vi "Kernel.vi"(0 "reference in":refnum<class "G#Object.lvclass">, 1 "object name":string, 2 "option 1":bool, 3 "option 2":bool, 4 "depth":i32, 5 "error in (no error)":errorcluster, 6 "state":T2, 7 "option 3":bool, 8 "attributes in":variant[](array[variant]), 10 "class attributes in":variant[](array[variant])) -> (11 "class attributes out":variant[](array[variant]), 12 "class hierarchy":T1[](array[typedef]), 13 "attributes out":variant[](array[variant]), 14 "reference out":refnum<class "G#Object.lvclass">, 15 "attribute refs":u32[](array[numeric]), 16 "static attribute ref":u32, 17 "output 1":bool, 18 "output 2":bool, 19 "error out":errorcluster)   [LabVIEW 2017, in "G#Object.lvclass"]
doc: "This is the G#object kernel that is responsible for creating and deleting object."
uses:
  G#Object.lvclass
  utils/G#Object_State.ctl
  utils/G#Object_ClassHierarchy.ctl
  G#Object.lvclass/G#Object.ctl
  utils/G#Object_ObjectInfoType.ctl
  utils/G#Object_CreateMethod.ctl
  utils/G#Object_EventType.ctl
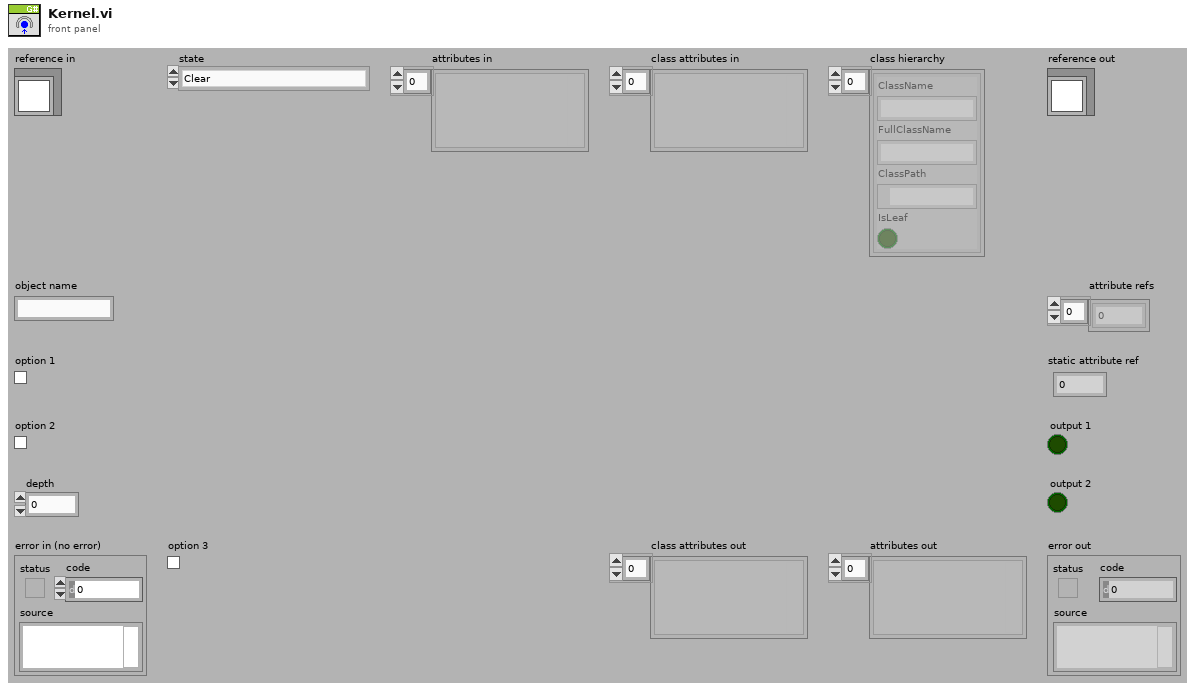
[diagram p1: front panel]
types:
  T1 = typedef "G#Object.lvclass/G#Object_ClassHierarchy.ctl" = cluster{"ClassName":string, "FullClassName":string, "ClassPath":path, "IsLeaf":bool}
  T2 = typedef "G#Object.lvclass/G#Object_State.ctl" = enum16{"Clear", "Create", "Delete", "Get class attributes", "Class hierarchy", "Get attribute value", "Set attribute value"}
  T3 = typedef "G#Object.lvclass/G#Object_ObjectInfoType.ctl" = cluster{"ObjectName":string, "ObjectID":u32, "Users":i32, "Counter":bool, "AttributeRefs":u32[], "FullClassName":string, "ClassName":string, "CreateMethod":T4, "GenericDestructorExists":bool, "Owner":string}
  T4 = typedef "G#Object.lvclass/G#Object_CreateMethod.ctl" = enum16{"Create", "Create or look up existing", "Look up existing"}
  T5 = typedef "G#Object.lvclass/G#Object_EventType.ctl" = enum16{"Created new", "Looked up existing", "Deleted", "Forced delete", "Not deleted", "Garbage collected", "Cleared", "User", "Error", "External create object", "External create class attributes", "Created class attributes", "Run constructor", "Run constructor done", "Run open method", "Run open method done"}
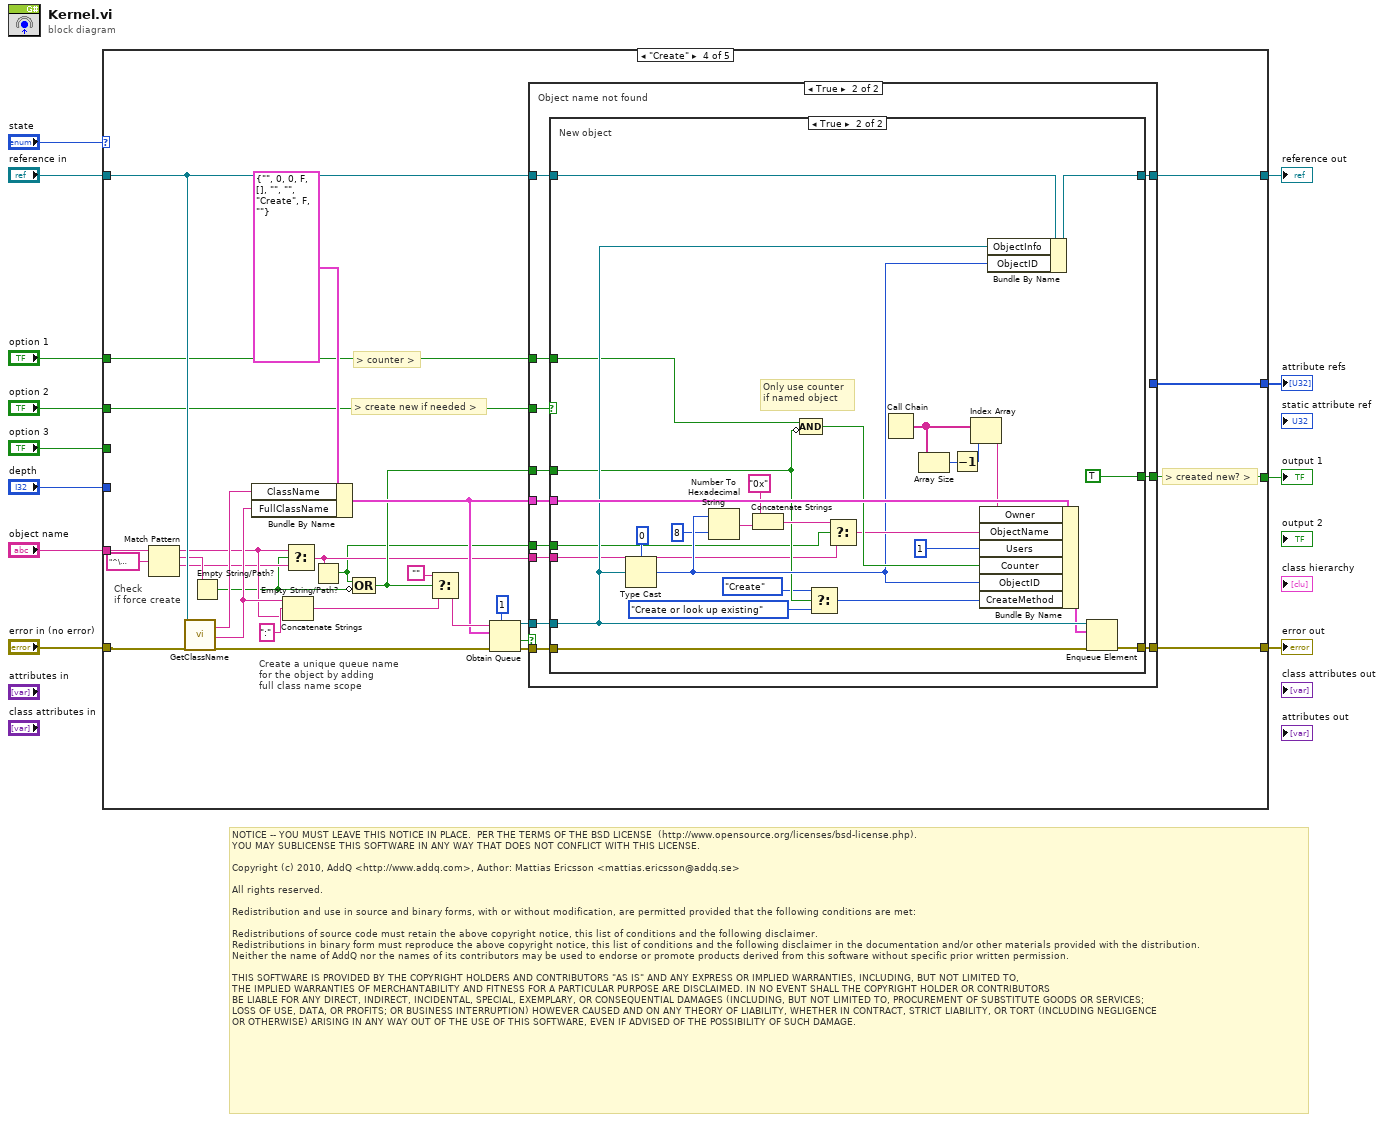
[diagram p0: block diagram]
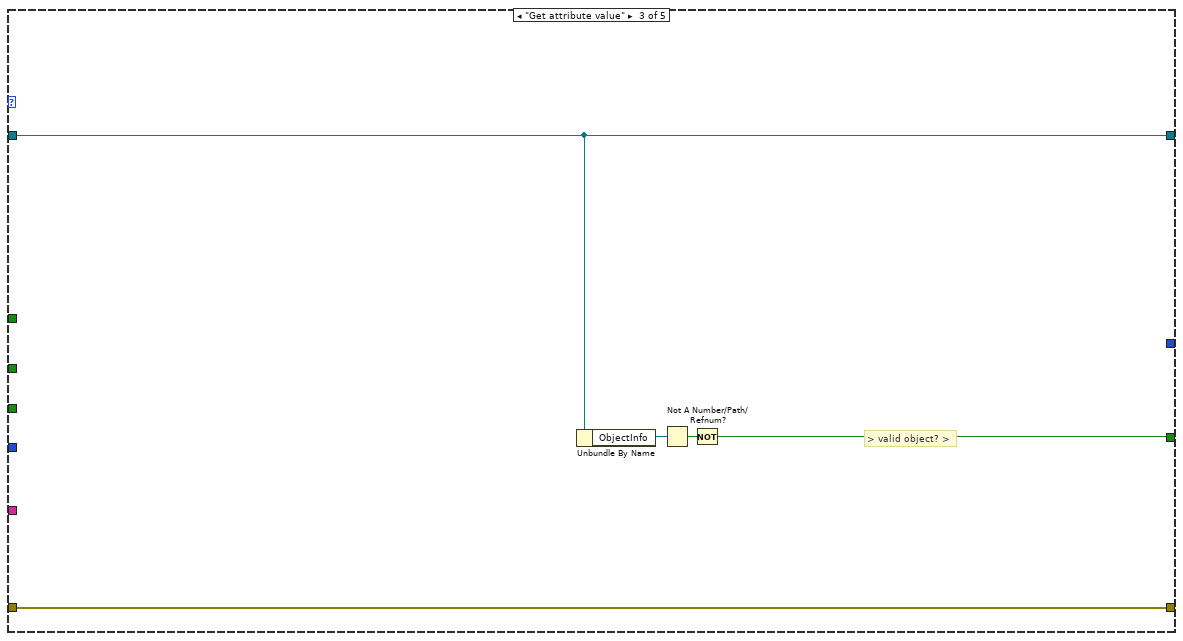
[diagram p4: hidden frame]
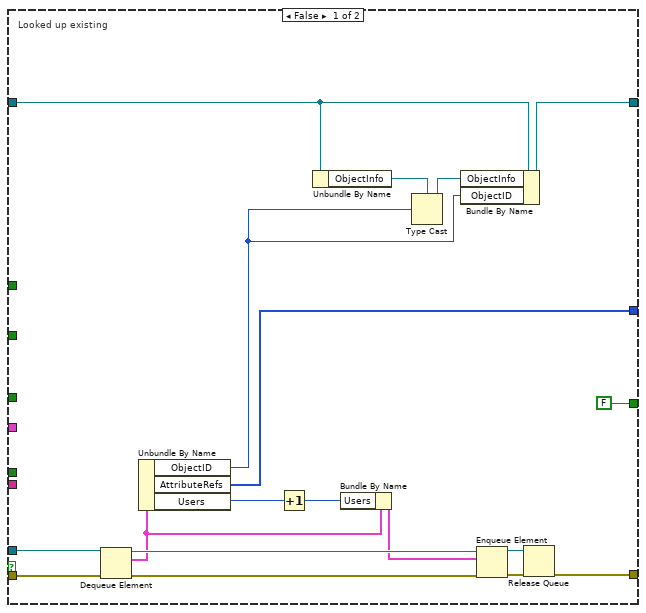
[diagram p5: hidden frame]
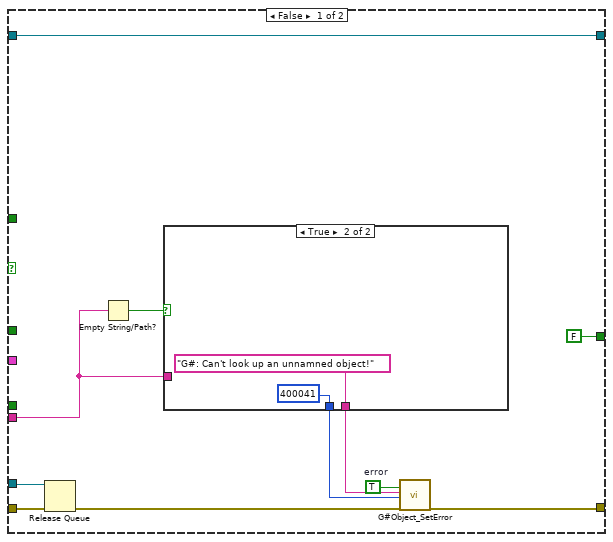
[diagram p6: hidden frame]
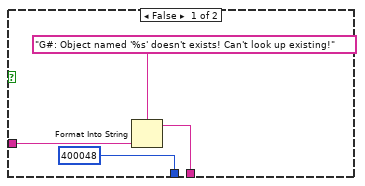
[diagram p7: hidden frame]
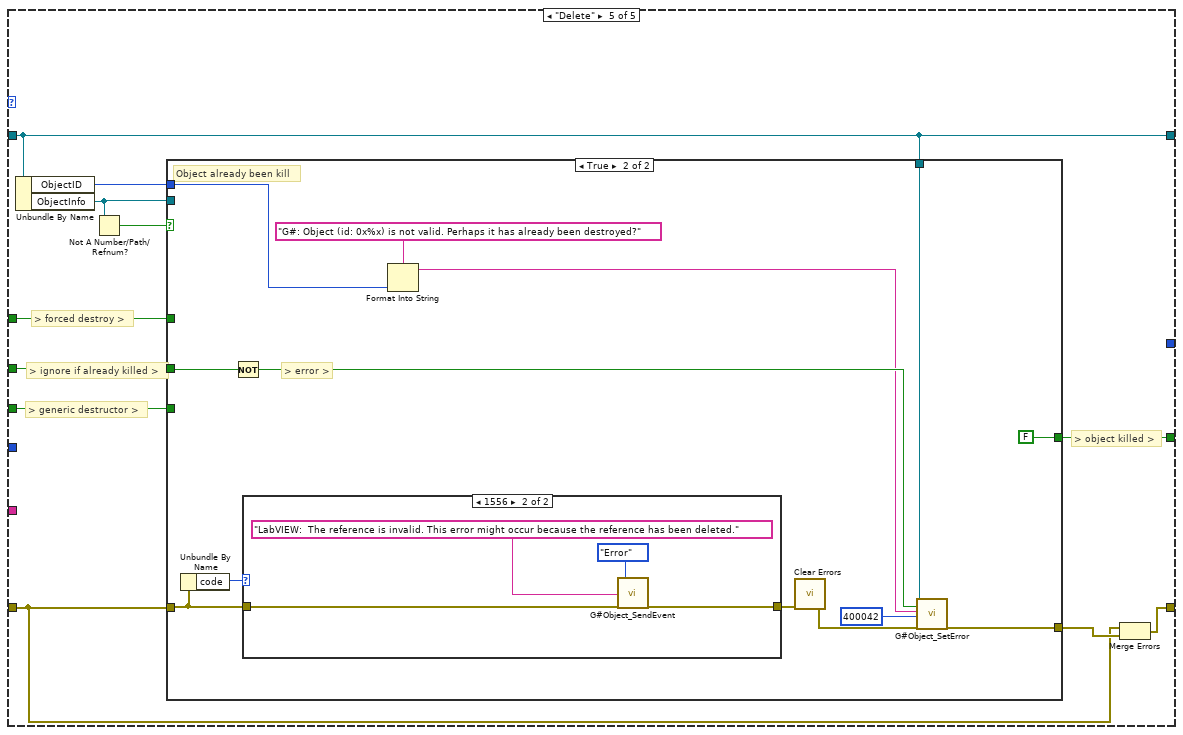
[diagram p8: hidden frame]
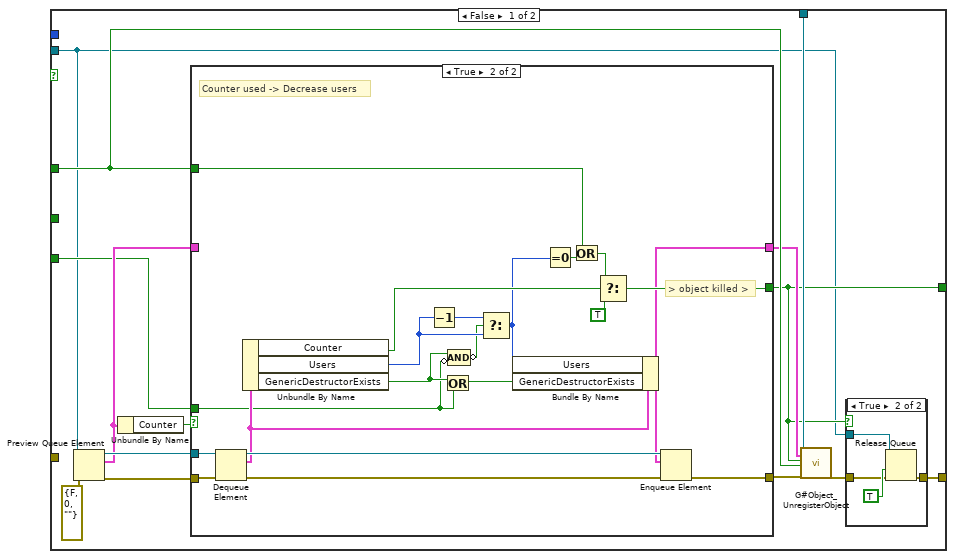
[diagram p9: hidden frame]
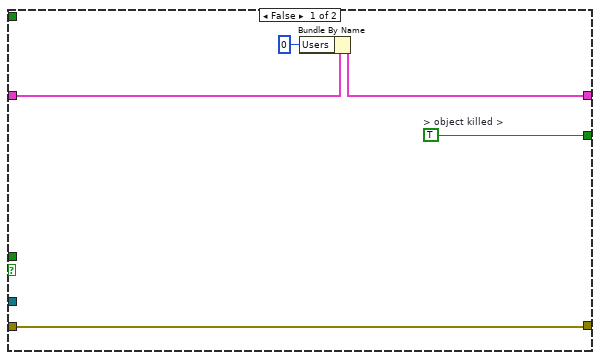
[diagram p11: hidden frame]
diagram:
  # "NOTICE -- YOU MUST LEAVE THIS NOTICE IN PLACE.  PER THE TERMS OF THE BSD LICENSE  (http://www.opensource.org/licenses/bsd-license.php).\nYOU MAY SUBLICENSE THIS SOFTWARE IN ANY WAY THAT DOES NOT CONFLICT WITH THIS LICENSE.\n\nCopyright (c) 2010, AddQ <http://www.addq.com>, Author: Mattias Ericsson <mattias.ericsson@addq.se>\n\nAll rights reserved.\n\nRedistribution and use in source and binary forms, with or without modification, are permitted provided that the following conditions are met:\n\nRedistributions of source code must retain the above copyright notice, this list of conditions and the following disclaimer.\nRedistributions in binary form must reproduce the above copyright notice, this list of conditions and the following disclaimer in the documentation and/or other materials provided with the distribution.\nNeither the name of AddQ nor the names of its contributors may be used to endorse or promote products derived from this software without specific prior written permission.\n \nTHIS SOFTWARE IS PROVIDED BY THE COPYRIGHT HOLDERS AND CONTRIBUTORS \"AS IS\" AND ANY EXPRESS OR IMPLIED WARRANTIES, INCLUDING, BUT NOT LIMITED TO,\nTHE IMPLIED WARRANTIES OF MERCHANTABILITY AND FITNESS FOR A PARTICULAR PURPOSE ARE DISCLAIMED. IN NO EVENT SHALL THE COPYRIGHT HOLDER OR CONTRIBUTORS\nBE LIABLE FOR ANY DIRECT, INDIRECT, INCIDENTAL, SPECIAL, EXEMPLARY, OR CONSEQUENTIAL DAMAGES (INCLUDING, BUT NOT LIMITED TO, PROCUREMENT OF SUBSTITUTE GOODS OR SERVICES;\nLOSS OF USE, DATA, OR PROFITS; OR BUSINESS INTERRUPTION) HOWEVER CAUSED AND ON ANY THEORY OF LIABILITY, WHETHER IN CONTRACT, STRICT LIABILITY, OR TORT (INCLUDING NEGLIGENCE\nOR OTHERWISE) ARISING IN ANY WAY OUT OF THE USE OF THIS SOFTWARE, EVEN IF ADVISED OF THE POSSIBILITY OF SUCH DAMAGE."
  n1 = case shown="\"Create\"" "state" {
    tunnel: "reference in" -> [w14 w16 w20 w37 w133]
    tunnel: [w14 w16 w20 w38 w133] -> w10
    tunnel: "error in (no error)" -> [w13 w15 w21 w42 w127]
    tunnel: [w13 w15 w21 w41 w136] -> w11
    tunnel: [_ _ w17 w33 w134] -> w8
    tunnel: [_ _ _ w39 _] -> w7
    tunnel: "option 1" -> [_ _ _ w36 w135]
    tunnel: "option 2" -> [_ _ _ w34 w131]
    tunnel: "object name" -> [_ _ _ w32 _]
    tunnel: "depth" -> [_ _ _ _ _]
    tunnel: "option 3" -> [_ _ _ _ w128]
    frame Default {
    }
    frame "Clear" {
      # "#ToDo Removed \"RequestDeallocation\" before NXG convert"
    }
    frame "Get attribute value" {
      # "> valid object? >"
      n2 = Unbundle By Name(w20) -> ("ObjectInfo"=w19:refnum<queue>)
      n3 = Not A Number/Path/Refnum?(number/path/refnum=w19) -> (NaN/Path/Refnum?=w18:bool)
      n4 = Not(x=w18) -> (.not. x?=w17:bool)
    }
    frame "Create" {
      # "Check\nif force create"
      # "> created new? >"
      # "> create new if needed >"
      # "> counter >"
      # "Create a unique queue name\nfor the object by adding\nfull class name scope"
      n5 = Match Pattern(string=w32, regular expression="^\u0000") -> (before substring=w27:string, match substring=w30:string, after substring=w26:string)  [unwired: 1 in, 1 out]
      n6 = call-dynamic "GetClassName.vi"("reference in"=w37, "error in (no error)"=w42) -> ("class name"=w43:string, "full class name"=w35:string, "error out"=w47:errorcluster)  [unwired: 13 in, 2 out]
      n7 = Empty String/Path?(string/path=w30) -> (empty?=w25:bool)
      n8 = Bundle By Name(cluster=T3 {"ObjectName"="", "ObjectID"=0, "Users"=0, "Counter"=FALSE, "AttributeRefs"=[], "FullClassName"="", "ClassName"="", "CreateMethod"=enum."Create", "GenericDestructorExists"=FALSE, "Owner"=""}, "ClassName"=w43, "FullClassName"=w35) -> (w44:T3)
      n9 = Concatenate Strings(w35, ":", w27) -> (w28:string)
      n10 = Select(t=w27, s=w25, f=w26) -> (s? t:f=w23:string)
      n11 = Empty String/Path?(string/path=w23) -> (empty?=w22:bool)
      n12 = Compound Arithmetic op=OR(w22, invert w25) -> (w24:bool)
      n13 = Select(t="", s=w24, f=w28) -> (s? t:f=w45:string)
      n14 = Obtain Queue(max queue size (-1, unlimited)=1, name (unnamed)=w45, element data type=w44, error in (no error)=w47) -> (queue out=w48:refnum<queue>, created new?=w40:bool, error out=w49:errorcluster)  [unwired: 1 in]
      n15 = case shown="True" w40 {
        tunnel: [w62 w81] -> w41
        tunnel: w49 -> [w69 w80]
        tunnel: w48 -> [w68 w76]
        tunnel: w44 -> [_ w79]
        tunnel: w37 -> [w59 w78]
        tunnel: [w58 w77] -> w38
        tunnel: [w56 _] -> w39
        tunnel: w36 -> [_ w75]
        tunnel: w24 -> [_ w74]
        tunnel: w23 -> [_ w73]
        tunnel: w34 -> [_ w72]
        tunnel: [FALSE w71] -> w33
        tunnel: w22 -> [_ w70]
        frame False {
          # "Looked up existing"
          n16 = Dequeue Element(queue=w68, error in (no error)=w69) -> (queue out=w66:refnum<queue>, element=w65:T3, error out=w67:errorcluster)  [unwired: 1 in, 1 out]
          n17 = Unbundle By Name(w65) -> ("ObjectID"=w54:u32, "AttributeRefs"=w56:u32[], "Users"=w64:i32)
          n18 = Increment(x=w64) -> (x+1=w52:i32)
          n19 = Unbundle By Name(w59) -> ("ObjectInfo"=w60:refnum<queue>)
          n20 = Bundle By Name(cluster=w65, "Users"=w52) -> (w55:T3)
          n21 = Type Cast(type=w60, x=w54) -> (*(type *) &x=w57:refnum<queue>)
          n22 = Bundle By Name(cluster=w59, "ObjectInfo"=w57, "ObjectID"=w54) -> (w58:refnum<class "G#Object.lvclass">)
          n23 = Enqueue Element(queue=w66, element=w55, error in (no error)=w67) -> (queue out=w61:refnum<queue>, error out=w63:errorcluster)  [unwired: 1 in, 1 out]
          n24 = Release Queue(queue=w61, error in (no error)=w63) -> (error out=w62:errorcluster)  [unwired: 1 in, 2 out]
        }
        frame True {
          # "Object name not found"
          n25 = case shown="True" w72 {
            tunnel: [w91 w126] -> w81
            tunnel: w80 -> [w85 w125]
            tunnel: w79 -> [_ w123]
            tunnel: w78 -> [w89 w121]
            tunnel: [w89 w120] -> w77
            tunnel: w76 -> [w83 w119]
            tunnel: w75 -> [_ w116]
            tunnel: w74 -> [_ w109]
            tunnel: w73 -> [w87 w100]
            tunnel: [FALSE TRUE] -> w71
            tunnel: w70 -> [_ w99]
            frame False {
              w90 = TRUE  # error
              n26 = Release Queue(queue=w83, error in (no error)=w85) -> (error out=w84:errorcluster)  [unwired: 1 in, 2 out]
              n27 = Empty String/Path?(string/path=w87) -> (empty?=w86:bool)
              n28 = case shown="True" w86 {
                tunnel: [w95 "G#: Can't look up an unnamned object!"] -> w88
                tunnel: w87 -> [w94 _]
                tunnel: [400048 ("code") 400041 ("code")] -> w82
                frame False {
                  n29 = Format Into String(format string="G#: Object named '%s' doesn't exists! Can't look up existing!", w94) -> (resulting string=w95:string)  [unwired: 2 in, 1 out]
                }
                frame True {
                }
              }
              n30 = call "G#Object_SetError.vi"("error (F)"=w90, "source"=w88, "code"=w82, "error in (no error)"=w84) -> ("error out"=w91:errorcluster)  [unwired: 15 in]
            }
            frame True {
              # "Only use counter\nif named object"
              # "New object"
              n31 = Type Cast(type=u32 0, x=w119) -> (*(type *) &x=w110:u32)
              n32 = Number To Hexadecimal String(1:i16 8 ("width (-)"), 2:w110) -> (0:w114:string)
              n33 = Concatenate Strings("0x" ("string"), w114) -> (w113:string)
              n34 = Compound Arithmetic op=AND(w116, invert w109) -> (w117:bool)
              n35 = Select(t=G#Object_CreateMethod."Create" ("CreateMethod"), s=w109, f=G#Object_CreateMethod."Create or look up existing" ("CreateMethod")) -> (s? t:f=w108:T4)
              n36 = Select(t=w113, s=w99, f=w100) -> (s? t:f=w115:string)
              n37 = Call Chain() -> (call chain=w103:string[])
              n38 = Array Size(array=w103) -> (size(s)=w102:i32)
              n39 = Decrement(x=w102) -> (x-1=w101:i32)
              n40 = Index Array(array=w103, index=w101) -> (element=w104:string)
              n41 = Bundle By Name(cluster=w123, "Owner"=w104, "ObjectName"=w115, "Users"=1, "Counter"=w117, "ObjectID"=w110, "CreateMethod"=w108) -> (w118:T3)
              n42 = Bundle By Name(cluster=w121, "ObjectInfo"=w119, "ObjectID"=w110) -> (w120:refnum<class "G#Object.lvclass">)
              n43 = Enqueue Element(queue=w119, element=w118, error in (no error)=w125) -> (error out=w126:errorcluster)  [unwired: 1 in, 2 out]
            }
          }
        }
      }
    }
    frame "Delete" {
      # "> generic destructor >"
      # "> ignore if already killed >"
      # "> object killed >"
      # "> forced destroy >"
      n44 = Unbundle By Name(w133) -> ("ObjectID"=w130:u32, "ObjectInfo"=w132:refnum<queue>)
      n45 = Not A Number/Path/Refnum?(number/path/refnum=w132) -> (NaN/Path/Refnum?=w129:bool)
      n46 = case shown="True" w129 {
        tunnel: w132 -> [w138 _]
        tunnel: [w140 w193] -> w137
        tunnel: w135 -> [w146 _]
        tunnel: [w139 FALSE ("f")] -> w134
        tunnel: w133 -> [w145 w187]
        tunnel: w131 -> [_ w192]
        tunnel: w130 -> [_ w191]
        tunnel: w128 -> [w142 _]
        tunnel: w127 -> [_ w185]
        frame False {
          n47 = Preview Queue Element(queue=w138, error in (no error)=errorcluster {"status"=FALSE, "code"=0, "source"=""}) -> (queue out=w149:refnum<queue>, element=w148:T3, error out=w150:errorcluster)  [unwired: 1 in, 1 out]
          n48 = Unbundle By Name(w148) -> ("Counter"=w151:bool)
          n49 = case shown="True" w151 {
            tunnel: [w157 w162] -> w144
            tunnel: w150 -> [w157 w172]
            tunnel: w149 -> [_ w173]
            tunnel: w146 -> [_ w177]
            tunnel: [w161 w175] -> w139
            tunnel: [w159 w170] -> w143
            tunnel: w148 -> [w160 _]
            tunnel: w142 -> [_ w164]
            frame False {
              w161 = TRUE  # > object killed >
              n50 = Bundle By Name(cluster=w160, "Users"=0) -> (w159:T3)
            }
            frame True {
              # "> object killed >"
              # "Counter used -> Decrease users"
              n51 = Dequeue Element(queue=w173, error in (no error)=w172) -> (queue out=w180:refnum<queue>, element=w171:T3, error out=w181:errorcluster)  [unwired: 1 in, 1 out]
              n52 = Unbundle By Name(w171) -> ("Counter"=w174:bool, "Users"=w166:i32, "GenericDestructorExists"=w165:bool)
              n53 = Decrement(x=w166) -> (x-1=w168:i32)
              n54 = Or(x=w165, y=w164) -> (x .or. y?=w169:bool)
              n55 = Compound Arithmetic op=AND(w165, invert w164) -> (invert w163:bool)
              n56 = Select(t=w168, s=w163, f=w166) -> (s? t:f=w167:i32)
              n57 = Bundle By Name(cluster=w171, "Users"=w167, "GenericDestructorExists"=w169) -> (w170:T3)
              n58 = Equal To 0?(x=w167) -> (x = 0?=w178:bool)
              n59 = Or(x=w177, y=w178) -> (x .or. y?=w176:bool)
              n60 = Select(t=w176, s=w174, f=TRUE) -> (s? t:f=w175:bool)
              n61 = Enqueue Element(queue=w180, element=w170, error in (no error)=w181) -> (error out=w162:errorcluster)  [unwired: 1 in, 2 out]
            }
          }
          n62 = call "G#Object_UnregisterObject.vi"("reference in"=w145, "object information"=w143, "object killed"=w139, "forced destroy"=w146, "error in (no error)"=w144) -> ("error out"=w141:errorcluster)  [unwired: 13 in, 1 out]
          n63 = case shown="True" w139 {
            tunnel: w141 -> [w152 w155]
            tunnel: [w152 w154] -> w140
            tunnel: w138 -> [_ w153]
            frame False {
            }
            frame True {
              n64 = Release Queue(queue=w153, force destroy? (F)=TRUE, error in (no error)=w155) -> (error out=w154:errorcluster)  [unwired: 2 out]
            }
          }
        }
        frame True {
          # "> error >"
          # "Object already been kill"
          n65 = Unbundle By Name(w185) -> ("code"=w186:i32)
          n66 = Not(x=w192) -> (.not. x?=w190:bool)
          n67 = case shown="1556" w186 {
            tunnel: w185 -> [w195 w198]
            tunnel: [w195 w197] -> w184
            frame 0, Default {
            }
            frame 1556 {
              n68 = call "G#Object_SendEvent.vi"("comment"="LabVIEW:  The reference is invalid. This error might occur because the reference has been deleted.", "error in (no error)"=w198, "G# event type"=G#Object_EventType."Error") -> ("error out"=w197:errorcluster)  [unwired: 16 in]
            }
          }
          n69 = Format Into String(format string="G#: Object (id: 0x%x) is not valid. Perhaps it has already been destroyed?" ("source"), w191) -> (resulting string=w188:string)  [unwired: 2 in, 1 out]
          n70 = call <vilib>:"Clear Errors.vi"("error in (no error)"=w184) -> ("error out"=w183:errorcluster)  [unwired: 5 in, 1 out]
          n71 = call "G#Object_SetError.vi"("reference in"=w187, "error (F)"=w190, "source"=w188, "code"=400042, "error in (no error)"=w183) -> ("error out"=w193:errorcluster)  [unwired: 14 in]
        }
      }
      n72 = Merge Errors(w127, w137) -> (w136:errorcluster)
    }
  }
  "error out" <- w11
  "reference out" <- w10
  "attribute refs" <- w7
  "output 1" <- w8
